vi "Read Id_c.vi"(11 "VISA resource name":refnum<visa-resource-name>="COM7") -> (2 "read string":string)   [LabVIEW 2017]
uses:
  controls/#typedef_Queue Cmd.ctl
panel:
  out "error out":errorcluster
  in  "error in (no error)":errorcluster
  in  "stop":bool
  in  "Get ID Button":bool
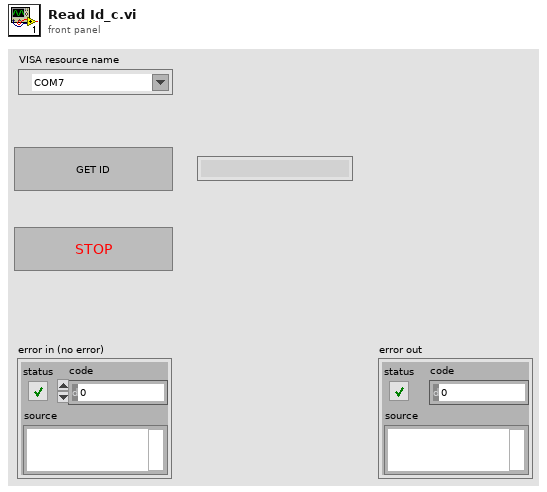
[diagram p1: front panel]
types:
  T1 = typedef "#typedef_Queue Cmd.ctl" = enum16{"Get ID", "Callib", "Go to", "Exit"}
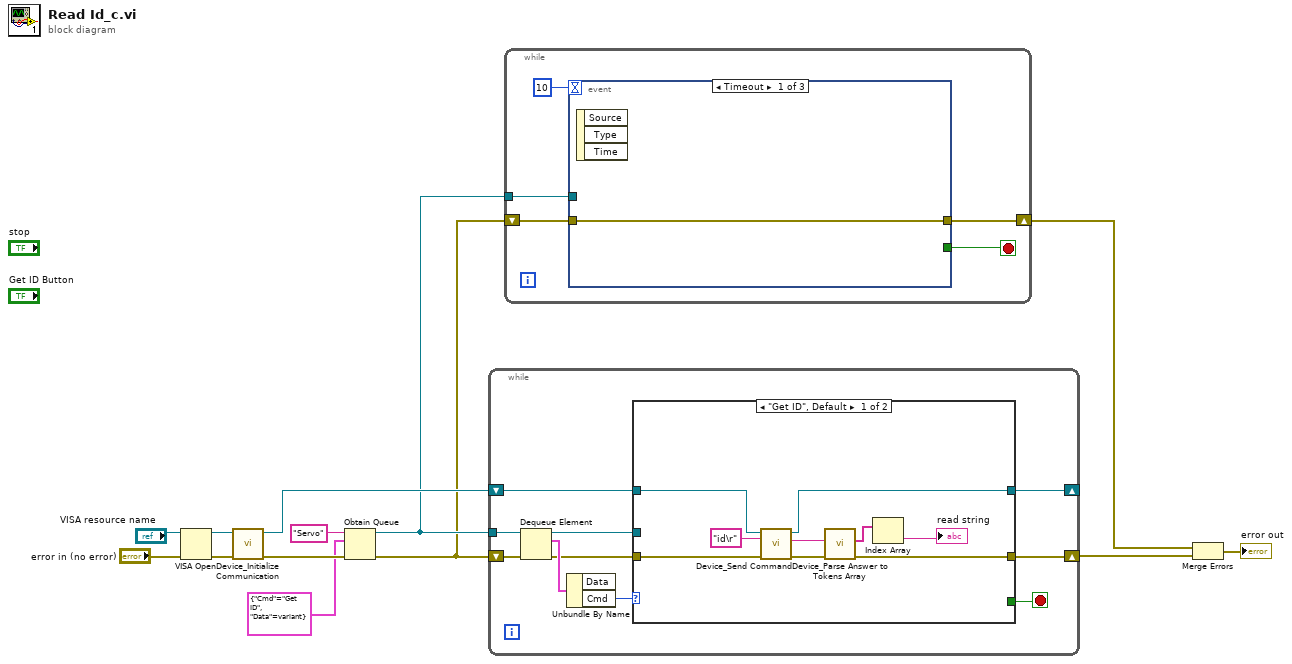
[diagram p0: block diagram]
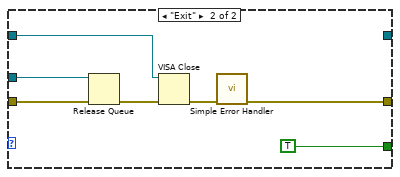
[diagram p2: hidden frame]
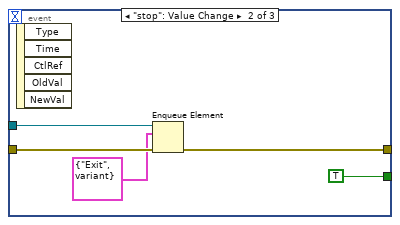
[diagram p3: hidden frame]
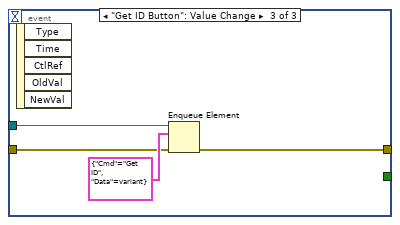
[diagram p4: hidden frame]
diagram:
  n1 = VISA Open(error in (no error)="error in (no error)", VISA resource name="VISA resource name") -> (VISA resource name=w12:refnum<visa-resource-name>, error out=w11:errorcluster)  [unwired: 3 in]
  n2 = call "Device_Initialize Communication.vi"("error in (no error)"=w11, "VISA Refnum in"=w12) -> ("error out"=w9:errorcluster, "VISA Refnum out"=w8:refnum<visa-resource-name>)  [unwired: 8 in]
  n3 = Obtain Queue(name (unnamed)="Servo", element data type=cluster{"Cmd":T1, "Data":variant} {"Cmd"=enum."Get ID", "Data"=variant} ("Queue Msg"), error in (no error)=w9) -> (queue out=w5:refnum<queue>, error out=w4:errorcluster)  [unwired: 2 in, 1 out]
  n4 = while {
    shift-right: [w14] -> _
    shift-left: w8 -> [w15]
    tunnel: w5 -> [w22]
    shift-right: [w17] -> w3
    shift-left: w4 -> [w23]
    stop <- w16 stop-if-true
    n5 = Dequeue Element(queue=w22, error in (no error)=w23) -> (queue out=w18:refnum<queue>, element=w21:cluster{"Cmd":T1, "Data":variant}, error out=w19:errorcluster)  [unwired: 1 in, 1 out]
    n6 = Unbundle By Name(w21) -> ("Cmd"=w20:T1)  [unwired: 1 out]
    n7 = case shown="\"Get ID\", Default" w20 {
      tunnel: w19 -> [w30 w39]
      tunnel: w18 -> [_ w38]
      tunnel: [w27 w33] -> w17
      tunnel: [_ TRUE] -> w16
      tunnel: w15 -> [w31 w35]
      tunnel: [w29 _] -> w14
      frame "Get ID", Default {
        n8 = call "Device_Send Command.vi"("error in (no error)"=w30, "write string"="id\r", "VISA Refnum in"=w31) -> ("error out"=w28:errorcluster, "read buffer"=w26:string, "VISA Refnum out"=w29:refnum<visa-resource-name>)  [unwired: 6 in]
        n9 = call "Device_Parse Answer to Tokens Array.vi"("error in (no error)"=w28, "Answer"=w26) -> ("error out"=w27:errorcluster, "Tokens Array"=w25:string[])  [unwired: 8 in]
        n10 = Index Array(array=w25) -> (element=→"read string":string)  [unwired: 1 in]
      }
      frame "Exit" {
        n11 = Release Queue(queue=w38, error in (no error)=w39) -> (error out=w34:errorcluster)  [unwired: 1 in, 2 out]
        n12 = VISA Close(VISA resource name=w35, error in (no error)=w34) -> (error out=w36:errorcluster)
        n13 = call <vilib>:"Simple Error Handler.vi"("error in (no error)"=w36) -> ("error out"=w33:errorcluster)  [unwired: 4 in, 4 out]
      }
    }
  }
  n14 = while {
    tunnel: w5 -> [w44]
    shift-right: [w42] -> w2
    shift-left: w4 -> [w43]
    stop <- w41 stop-if-true
    n15 = event shown="[0] Timeout" {
      selector: _ -> [_ _ _]
      dyn-events: _ -> [_ _ _]
      timeout: 10 -> [_ _ _]
      tunnel: w44 -> [_ w47 w52]
      tunnel: w43 -> [w45 w50 w53]
      tunnel: [w45 w49 w51] -> w42
      tunnel: [_ TRUE _] -> w41
      event Timeout {
        n16 = event-data() -> ()  [unwired: 1 in, 3 out]
      }
      event "stop": Value Change {
        n17 = event-data() -> ()  [unwired: 1 in, 5 out]
        n18 = Enqueue Element(queue=w47, element=cluster{"Cmd":T1, "Data":variant} {"Cmd"=enum."Exit", "Data"=variant} ("Queue Msg"), error in (no error)=w50) -> (error out=w49:errorcluster)  [unwired: 1 in, 2 out]
      }
      event "Get ID Button": Value Change {
        n19 = event-data() -> ()  [unwired: 1 in, 5 out]
        n20 = Enqueue Element(queue=w52, element=cluster{"Cmd":T1, "Data":variant} {"Cmd"=enum."Get ID", "Data"=variant} ("Queue Msg"), error in (no error)=w53) -> (error out=w51:errorcluster)  [unwired: 1 in, 2 out]
      }
    }
  }
  n21 = Merge Errors(w2, w3) -> (→"error out":errorcluster)
